vi "Begin.vi"() -> (1 "CameraDevRef":T5)   [LabVIEW 2011]
doc: "Called before other user functions, this VI is expected to open initial I/O refnums, load in file data, and do all program initialization. Notice that the <B>error out</B> terminal is simply used for data flow. Wiring it to other structures or subVIs ensures that this VI runs first."
uses:
  <vilib>/Rock Robotics/WPI/Camera/WPI_CameraDevRef.ctl
  <vilib>/Rock Robotics/WPI/Encoder/WPI_EncoderDevRef.ctl
  <vilib>/Rock Robotics/SystemInterfaces/Encoder/FPGA_EncoderIdx.ctl
  <vilib>/Rock Robotics/SystemInterfaces/Counter/FPGA_CounterCtrSystemIndex.ctl
  <vilib>/Rock Robotics/WPI/Encoder/WPI_EncoderType.ctl
  <vilib>/Rock Robotics/WPI/Joystick/WPI_JoystickDeviceEnum.ctl
  <vilib>/Rock Robotics/SystemInterfaces/DIO/FPGA_DIOPWMChannel.ctl
  <vilib>/Rock Robotics/SystemInterfaces/Typedef/FPGA_TypedefDigitalModule.ctl
  <vilib>/Rock Robotics/WPI/MotorControl/WPI_MotorControlOpen Victor.vi
  Robot Global Data.vi
  <vilib>/Rock Robotics/SystemInterfaces/DIO/FPGA_DIORelayChannel.ctl
  <vilib>/Rock Robotics/WPI/Relay/WPI_RelayDirection.ctl
  <vilib>/Rock Robotics/SystemInterfaces/AI/FPGA_AIChannel.ctl
  <vilib>/Rock Robotics/WPI/Counter/WPI_CounterDigitalInputToDigitalSource.vi
  <vilib>/Rock Robotics/SystemInterfaces/DIO/FPGA_DIOChannel.ctl
  <vilib>/Rock Robotics/SystemInterfaces/AI/FPGA_AIGyroChannel.ctl
  <vilib>/Rock Robotics/WPI/MotorControl/WPI_MotorControlOpen Jaguar.vi
  <vilib>/Rock Robotics/SystemInterfaces/Typedef/FPGA_TypedefAnalogModule.ctl
  <vilib>/Utility/file.llb/Read From Spreadsheet File (DBL).vi
panel:
  in  "Balls In Robot At Start":dbl=2.0
  out "LDriveEncoder 3":cluster{"status":bool}
  out "EncoderDevRef 3":T1={"DevStatus"={"status"=FALSE, "code"=0, "source"=""}, "EncoderIndex"=enum."Invalid", "CounterIndex"=enum."Invalid", "DistancePerCount"=1.0, "Decoding Type"=enum."4x"}
  out "EncoderDevRef 2":T1={"DevStatus"={"status"=FALSE, "code"=0, "source"=""}, "EncoderIndex"=enum."Invalid", "CounterIndex"=enum."Invalid", "DistancePerCount"=1.0, "Decoding Type"=enum."4x"}
  out "LDriveEncoder 2":errorcluster
  out "EncoderDevRef":T1={"DevStatus"={"status"=FALSE, "code"=0, "source"=""}, "EncoderIndex"=enum."Invalid", "CounterIndex"=enum."Invalid", "DistancePerCount"=1.0, "Decoding Type"=enum."4x"}
  out "LDriveEncoder":errorcluster
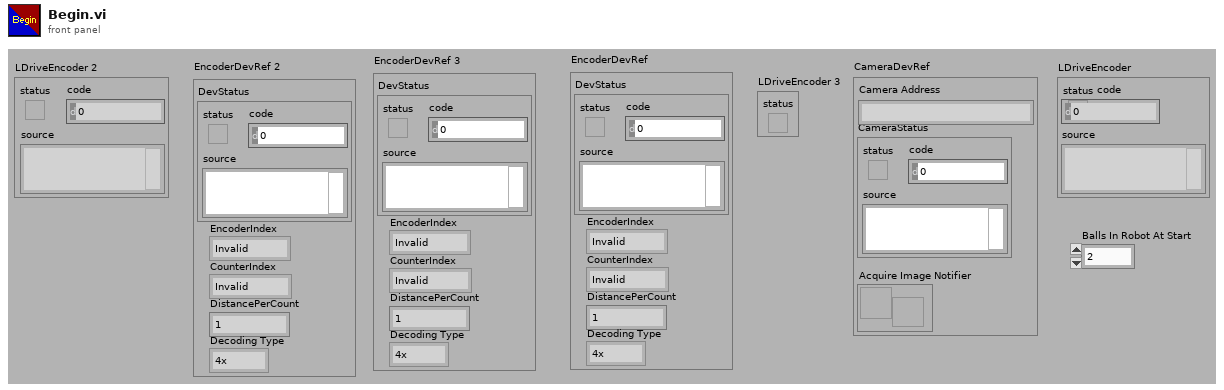
[diagram p1: front panel]
types:
  T1 = typedef "WPI_EncoderDevRef.ctl" = cluster{"DevStatus":errorcluster, "EncoderIndex":T2, "CounterIndex":T3, "DistancePerCount":dbl, "Decoding Type":T4}
  T2 = typedef "FPGA_EncoderIdx.ctl" = enum8{"Enc 0", "Enc 1", "Enc 2", "Enc 3", "Invalid"}
  T3 = typedef "FPGA_CounterCtrSystemIndex.ctl" = enum8{"Ctr 0", "Ctr 1", "Ctr 2", "Ctr 3", "Ctr 4", "Ctr 5", "Ctr 6", "Ctr 7", "Invalid"}
  T4 = typedef "WPI_EncoderType.ctl" = enum16{"1x", "2x", "4x"}
  T5 = typedef "WPI_CameraDevRef.ctl" = cluster{"Camera Address":string, "CameraStatus":errorcluster, "Acquire Image Notifier":refnum<notifier>}
  T6 = typedef "FPGA_TypedefDigitalModule.ctl" = enum16{"Digital Module 1", "Digital Module 2"}
  T7 = typedef "FPGA_DIOPWMChannel.ctl" = enum8{"PWM 1", "PWM 2", "PWM 3", "PWM 4", "PWM 5", "PWM 6", "PWM 7", "PWM 8", "PWM 9", "PWM 10", "Invalid"}
  T8 = typedef "WPI_JoystickDeviceEnum.ctl" = enum16{"USB 1", "USB 2", "USB 3", "USB 4", "Kinect 1", "Kinect 2"}
  T9 = typedef "FPGA_DIORelayChannel.ctl" = enum8{"Relay 1", "Relay 2", "Relay 3", "Relay 4", "Relay 5", "Relay 6", "Relay 7", "Relay 8", "Invalid"}
  T10 = typedef "FPGA_AIChannel.ctl" = enum8{"AI 1", "AI 2", "AI 3", "AI 4", "AI 5", "AI 6", "AI 7", "AI 8", "Invalid"}
  T11 = typedef "WPI_RelayDevRef.ctl" = cluster{"DevStatus":errorcluster, "Relay Channel":T9, "Digital Module":T6, "Relay Direction":T12}
  T12 = typedef "WPI_RelayDirection.ctl" = enum16{"Both directions", "Forward only", "Reverse only"}
  T13 = typedef "WPI_AnalogChannelDevRef.ctl" = cluster{"DevStatus":errorcluster, "Analog Module":T14, "Analog Channel":T10}
  T14 = typedef "FPGA_TypedefAnalogModule.ctl" = enum16{"Analog Module 1", "Analog Module 2"}
  T15 = typedef "WPI_MotorControlDeviceRef.ctl" = cluster{"DeviceStatus":errorcluster, "Type":enum16{"PWM", "CAN"}, "PWM":cluster{"Digital Module":T6, "PWM Channel":T7, "DeadBand":T16}, "CAN":cluster{"Device Number":u8, "Control Mode":T17, "Semaphore":T18, "Max Vout":dbl}, "Invert":bool, "TransformRef":T19, "InvTransformRef":T19}
  T16 = typedef "WPI_PWMDeadband.ctl" = cluster{"Name":string, "maxPositivePwm":i32, "minPositivePwm":i32, "centerPwm":i32, "maxNegativePwm":i32, "minNegativePwm":i32, "angularRange":u16}
  T17 = typedef "WPI_CANJaguar_ControlMode.ctl" = enum8{"Percent VBus", "Current", "Speed", "Position", "Voltage"}
  T18 = typedef "Semaphore RefNum" = refnum<k1>
  T19 = typedef "WPI_PWMTransform_ConPane.ctl" = refnum<vi>
  T20 = typedef "WPI_CameraImageSize.ctl" = enum16{"640x480", "320x240", "160x120"}
  T21 = cluster{"fps":i32, "compression":i32, "Image Size":T20}
  T22 = typedef "WPI_CameraWhite Balance Values.ctl" = enum16{"Auto", "Fixed indoor", "Fixed outdoor 1", "Fixed outdoor 2", "Fixed fluorescent 1", "Fixed fluorescent 2", "Hold current"}
  T23 = typedef "WPI_CameraExposure Values.ctl" = enum16{"Auto", "Flicker-free 50 Hz", "Flicker-free 60 Hz", "Hold current"}
  T24 = typedef "WPI_ServoDeviceRef.ctl" = cluster{"DeviceStatus":errorcluster, "Digital Module":T6, "PWM Channel":T7, "DeadBand":T16}
  T25 = typedef "FPGA_DIOChannel.ctl" = enum8{"DIO 1", "DIO 2", "DIO 3", "DIO 4", "DIO 5", "DIO 6", "DIO 7", "DIO 8", "DIO 9", "DIO 10", "DIO 11", "DIO 12", "DIO 13", "DIO 14", "Invalid"}
  T26 = typedef "WPI_DigitalInputDevRef.ctl" = cluster{"DevStatus":errorcluster, "DIO Channel":T25, "Digital Module":T6}
  T27 = typedef "FPGA_CounterEncoderSourceConvertionLVSourceType.ctl" = cluster{"DevStatus":errorcluster, "AnalogTriggerMode?":bool, "DigitalMode":cluster{"Digital Module":T6, "DIO Channel":T28}, "AnalogTriggerMode":cluster{"AnalogTriggerIndex":T29, "OutputType":T30}}
  T28 = typedef "FPGA_DIODigitalSourceChannel.ctl" = enum8{"DIO 1", "DIO 2", "DIO 3", "DIO 4", "DIO 5", "DIO 6", "DIO 7", "DIO 8", "DIO 9", "DIO 10", "DIO 11", "DIO 12", "DIO 13", "DIO 14", "Disabled"}
  T29 = typedef "FPGA_AnalogTriggerIndex.ctl" = enum8{"Trig 0", "Trig 1", "Trig 2", "Trig 3", "Trig 4", "Trig 5", "Trig 6", "Trig 7", "Invalid"}
  T30 = typedef "FPGA_AnalogTriggerOutType.ctl" = enum16{"InWindow", "TriggerState", "Rising", "Falling"}
  T31 = typedef "WPI_JoystickDevRef.ctl" = cluster{"Device":T8}
  T32 = typedef "FPGA_AIGyroChannel.ctl" = enum8{"AI 1", "AI 2", "Invalid"}
  T33 = typedef "WPI_GyroDevRef.ctl" = cluster{"DevStatus":errorcluster, "Analog Module":T14, "Analog Channel":T10, "Offset":dbl, "Gain (VoltsPerDegree/Second)":dbl}
  T34 = typedef "WPI_UltrasonicDeviceRef.ctl" = cluster{"DevStatus":errorcluster, "Ping Digital Module":T6, "Echo Digital Module":T6, "Ping Channel":T25, "Echo Channel":T25, "CntIndex":T3}
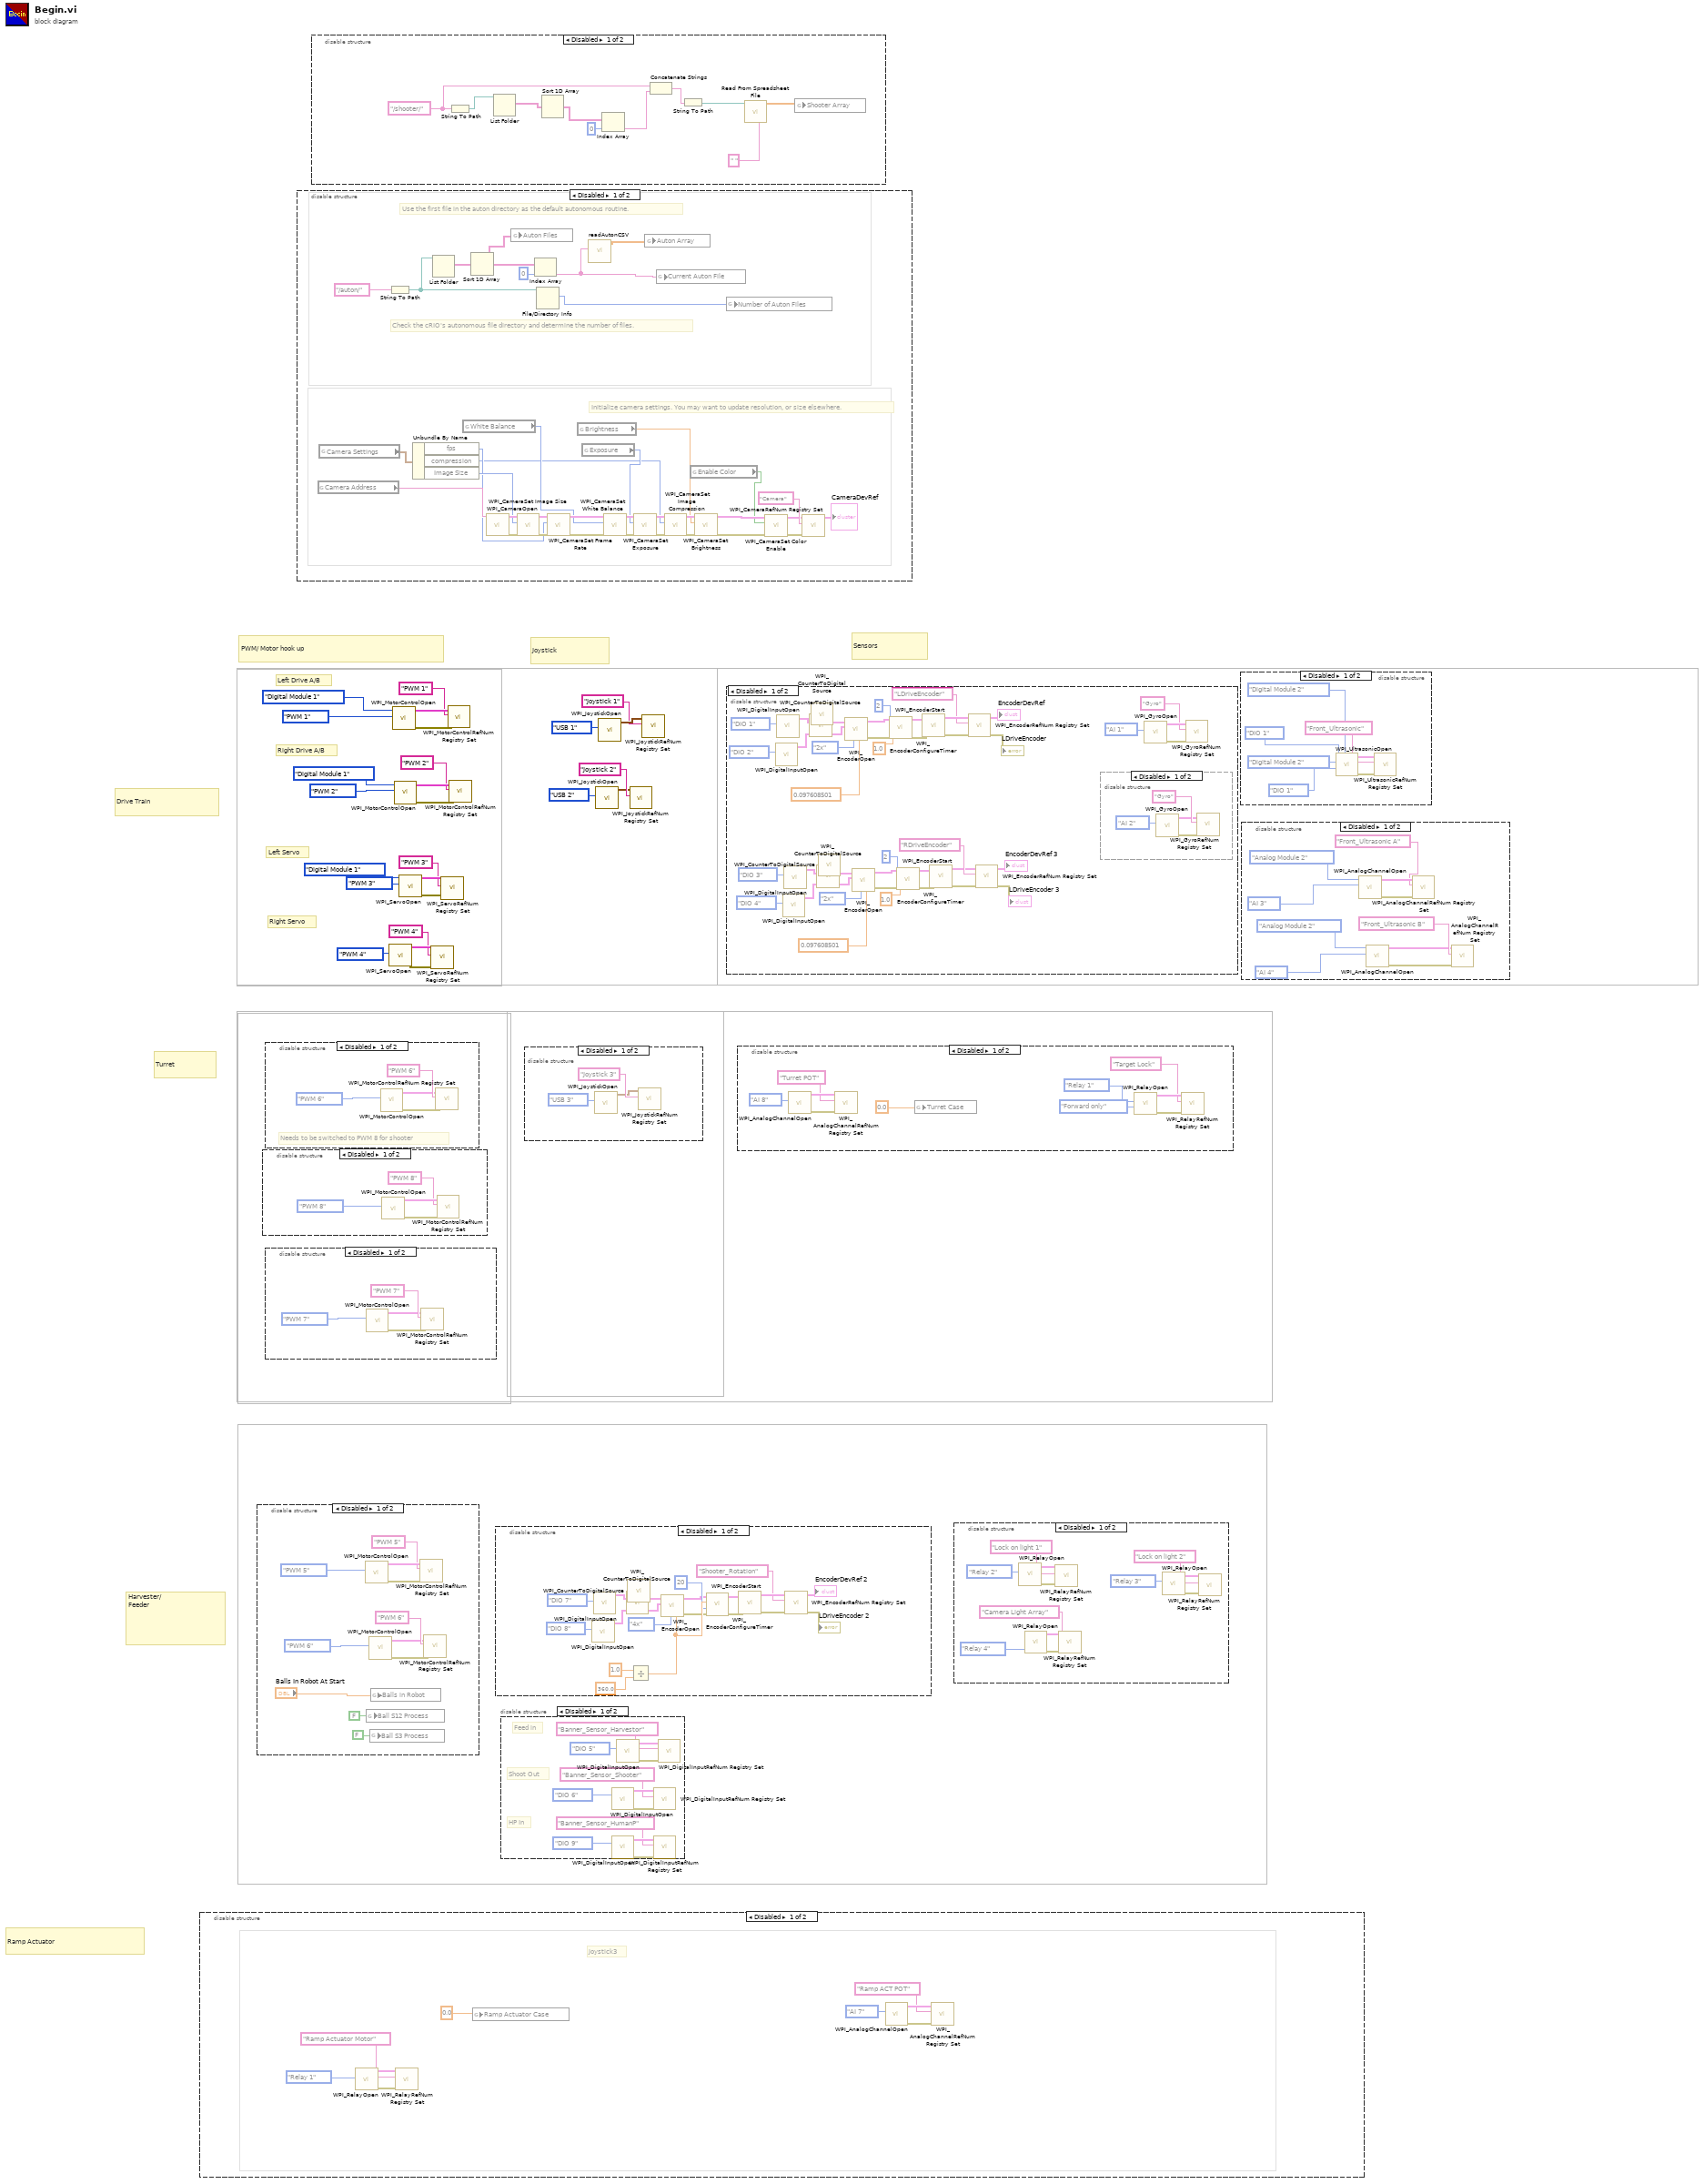
[diagram p0: block diagram]
diagram:
  # "Harvester/\nFeeder"
  # "Right Drive A/B"
  # "Left Drive A/B"
  # "Right Servo"
  # "Left Servo"
  # "Turret"
  # "Ramp Actuator"
  # "Drive Train"
  # "Sensors"
  # "Joystick"
  # "PWM/ Motor hook up"
  n1 = disable-structure shown="Disabled" {
    frame Disabled {
      # "Joystick3"
      n2 = call <vilib>:"WPI_RelayOpen.vi"("Relay Channel"=FPGA_DIORelayChannel."Relay 1") -> ("error out"=w30:errorcluster, "RelayDevRef"=w29:T11)  [unwired: 9 in]
      n3 = call <vilib>:"WPI_RelayRefNum Registry Set.vi"("error in (no error)"=w30, "refnum name"="Ramp Actuator Motor", "RelayDevRef"=w29) -> ()  [unwired: 7 in, 2 out]
      n4 = global write "Robot Global Data.vi" "Ramp Actuator Case"(0.0 ("Ramp Actuator Case")) -> ()
      n5 = call <vilib>:"WPI_AnalogChannelOpen.vi"("Analog Channel"=FPGA_AIChannel."AI 7") -> ("error out"=w33:errorcluster, "AIDeviceRef"=w34:T13)  [unwired: 9 in]
      n6 = call <vilib>:"WPI_AnalogChannelRefNum Registry Set.vi"("error in (no error)"=w33, "refnum name"="Ramp ACT POT", "AIDeviceRef"=w34) -> ()  [unwired: 7 in, 2 out]
    }
    frame Enabled {
    }
  }
  n7 = disable-structure shown="Disabled" {
    frame Disabled {
      n8 = call-poly <vilib>:"WPI_MotorControlOpen.vi"("PWM Channel"=FPGA_DIOPWMChannel."PWM 5") -> ("error out"=w42:errorcluster, "MotorControlDeviceRef"=w44:T15)  [unwired: 9 in]
      n9 = global write "Robot Global Data.vi" "Ball S12 Process"(FALSE ("Ball S12 Process")) -> ()
      n10 = call-poly <vilib>:"WPI_MotorControlOpen.vi"("PWM Channel"=FPGA_DIOPWMChannel."PWM 6") -> ("error out"=w41:errorcluster, "MotorControlDeviceRef"=w39:T15)  [unwired: 9 in]
      n11 = global write "Robot Global Data.vi" "Ball S3 Process"(FALSE ("Ball S3 Process")) -> ()
      n12 = global write "Robot Global Data.vi" "Balls in Robot"("Balls In Robot At Start") -> ()
      n13 = call <vilib>:"WPI_MotorControlRefNum Registry Set.vi"("error in (no error)"=w42, "refnum name"="PWM 5", "MotorControlDevRef"=w44) -> ()  [unwired: 7 in, 2 out]
      n14 = call <vilib>:"WPI_MotorControlRefNum Registry Set.vi"("error in (no error)"=w41, "refnum name"="PWM 6", "MotorControlDevRef"=w39) -> ()  [unwired: 7 in, 2 out]
    }
    frame Enabled {
    }
  }
  n15 = disable-structure shown="Disabled" {
    frame Disabled {
      n16 = call-poly <vilib>:"WPI_MotorControlOpen.vi"("PWM Channel"=FPGA_DIOPWMChannel."PWM 8") -> ("error out"=w46:errorcluster, "MotorControlDeviceRef"=w48:T15)  [unwired: 9 in]
      n17 = call <vilib>:"WPI_MotorControlRefNum Registry Set.vi"("error in (no error)"=w46, "refnum name"="PWM 8", "MotorControlDevRef"=w48) -> ()  [unwired: 7 in, 2 out]
    }
    frame Enabled {
    }
  }
  n18 = disable-structure shown="Disabled" {
    frame Disabled {
      # "Needs to be switched to PWM 8 for shooter"
      n19 = call-poly <vilib>:"WPI_MotorControlOpen.vi"("PWM Channel"=FPGA_DIOPWMChannel."PWM 6") -> ("error out"=w53:errorcluster, "MotorControlDeviceRef"=w51:T15)  [unwired: 9 in]
      n20 = call <vilib>:"WPI_MotorControlRefNum Registry Set.vi"("error in (no error)"=w53, "refnum name"="PWM 6", "MotorControlDevRef"=w51) -> ()  [unwired: 7 in, 2 out]
    }
    frame Enabled {
    }
  }
  n21 = disable-structure shown="Disabled" {
    frame Disabled {
      n22 = call-poly <vilib>:"WPI_MotorControlOpen.vi"("PWM Channel"=FPGA_DIOPWMChannel."PWM 7") -> ("error out"=w57:errorcluster, "MotorControlDeviceRef"=w55:T15)  [unwired: 9 in]
      n23 = call <vilib>:"WPI_MotorControlRefNum Registry Set.vi"("error in (no error)"=w57, "refnum name"="PWM 7", "MotorControlDevRef"=w55) -> ()  [unwired: 7 in, 2 out]
    }
    frame Enabled {
    }
  }
  n24 = disable-structure shown="Disabled" {
    frame Disabled {
      # "Check the cRIO's autonomous file directory and determine the number of files."
      # "Use the first file in the auton directory as the default autonomous routine."
      # "Initialize camera settings. You may want to update resolution, or size elsewhere."
      n25 = global read "Robot Global Data.vi" "Camera Address"() -> (w79:string)
      n26 = global read "Robot Global Data.vi" "Camera Settings"() -> (w78:T21)
      n27 = String To Path(string="/auton/") -> (path=w64:path)
      n28 = Unbundle By Name(w78) -> ("fps"=w76:i32, "compression"=w73:i32, "Image Size"=w77:T20)
      n29 = List Folder(path=w64) -> (filenames=w63:string[])  [unwired: 1 in, 5 out]
      n30 = global read "Robot Global Data.vi" "White Balance"() -> (w75:T22)
      n31 = Sort 1D Array(array=w63) -> (sorted array=w58:string[])
      n32 = call <vilib>:"WPI_CameraOpen.vi"("Camera Address"=w79) -> ("error out"=w85:errorcluster, "CameraDevRef"=w86:T5)  [unwired: 1 in, 8 out]
      n33 = global write "Robot Global Data.vi" "Auton Files"(w58) -> ()
      n34 = call <vilib>:"WPI_CameraSet Image Size.vi"("error in (no error)"=w85, "Image Size"=w77, "CameraDevRef"=w86) -> ("error out"=w84:errorcluster, "CameraDevRef Out"=w87:T5)  [unwired: 7 out]
      n35 = Index Array(array=w58, index=0) -> (element=w60:string)
      n36 = File/Directory Info(path=w64) -> (size=w61:i64)  [unwired: 1 in, 6 out]
      n37 = call <vilib>:"WPI_CameraSet Frame Rate.vi"("error in (no error)"=w84, "Frame Rate (fps)"=w76, "CameraDevRef"=w87) -> ("error out"=w83:errorcluster, "CameraDevRef Out"=w89:T5)  [unwired: 7 out]
      n38 = global read "Robot Global Data.vi" "Brightness"() -> (w72:dbl)
      n39 = global read "Robot Global Data.vi" "Exposure"() -> (w74:T23)
      n40 = call "readAutonCSV.vi"("AutonFile"=w60) -> ("AutonArray"=w59:dbl[][])  [unwired: 7 in]
      n41 = call <vilib>:"WPI_CameraSet White Balance.vi"("error in (no error)"=w83, "White Balance"=w75, "CameraDevRef"=w89) -> ("error out"=w82:errorcluster, "CameraDevRef Out"=w88:T5)  [unwired: 7 out]
      n42 = call <vilib>:"WPI_CameraSet Exposure.vi"("error in (no error)"=w82, "Exposure"=w74, "CameraDevRef"=w88) -> ("error out"=w81:errorcluster, "CameraDevRef Out"=w91:T5)  [unwired: 7 out]
      n43 = global write "Robot Global Data.vi" "Auton Array"(w59) -> ()
      n44 = global write "Robot Global Data.vi" "Current Auton File"(w60) -> ()
      n45 = call <vilib>:"WPI_CameraSet Image Compression.vi"("error in (no error)"=w81, "Compression"=w73, "CameraDevRef"=w91) -> ("error out"=w80:errorcluster, "CameraDevRef Out"=w90:T5)  [unwired: 7 out]
      n46 = global read "Robot Global Data.vi" "Enable Color"() -> (w67:bool)
      n47 = call <vilib>:"WPI_CameraSet Brightness.vi"("error in (no error)"=w80, "Brightness"=w72, "CameraDevRef"=w90) -> ("error out"=w70:errorcluster, "CameraDevRef Out"=w71:T5)  [unwired: 7 out]
      n48 = global write "Robot Global Data.vi" "Number of Auton Files"(w61) -> ()
      n49 = call <vilib>:"WPI_CameraSet Color Enable.vi"("error in (no error)"=w70, "Color Enabled"=w67, "CameraDevRef"=w71) -> ("error out"=w68:errorcluster, "CameraDevRef Out"=w69:T5)  [unwired: 7 in]
      n50 = call <vilib>:"WPI_CameraRefNum Registry Set.vi"("error in (no error)"=w68, "refnum name"="Camera", "CameraDevRef"=w69) -> ("CameraDevRef"=→"CameraDevRef":T5)  [unwired: 8 out]
    }
    frame Enabled {
    }
  }
  n51 = disable-structure shown="Disabled" {
    frame Disabled {
      w101 = "/shooter/" ("string")
      n52 = String To Path(string=w101) -> (path=w102:path)
      n53 = List Folder(path=w102) -> (filenames=w100:string[])  [unwired: 1 in, 5 out]
      n54 = Sort 1D Array(array=w100) -> (sorted array=w99:string[])
      n55 = Index Array(array=w99, index=0) -> (element=w97:string)
      n56 = Concatenate Strings(w101, w97) -> (w96:string)
      n57 = String To Path(string=w96) -> (path=w95:path)
      n58 = call-poly <vilib>:"Read From Spreadsheet File.vi"("delimiter (\\t)"=" " ("delimiter (\\t)"), "file path (dialog if empty)"=w95) -> ("all rows"=w93:dbl[][])  [unwired: 5 in, 4 out]
      n59 = global write "Robot Global Data.vi" "Shooter Array"(w93) -> ()
    }
    frame Enabled {
    }
  }
  n60 = call <vilib>:"WPI_ServoOpen.vi"("PWM Channel"=FPGA_DIOPWMChannel."PWM 4") -> ("error out"=w1:errorcluster, "ServoDeviceRef"=w16:T24)  [unwired: 9 in]
  n61 = call-poly <vilib>:"WPI_MotorControlOpen.vi"("PWM Channel"=FPGA_DIOPWMChannel."PWM 1", "Digital Module (Module 1)"=FPGA_TypedefDigitalModule."Digital Module 1") -> ("error out"=w6:errorcluster, "MotorControlDeviceRef"=w9:T15)  [unwired: 8 in]
  n62 = call-poly <vilib>:"WPI_MotorControlOpen.vi"("PWM Channel"=FPGA_DIOPWMChannel."PWM 2", "Digital Module (Module 1)"=FPGA_TypedefDigitalModule."Digital Module 1") -> ("error out"=w7:errorcluster, "MotorControlDeviceRef"=w12:T15)  [unwired: 8 in]
  n63 = call <vilib>:"WPI_ServoOpen.vi"("PWM Channel"=FPGA_DIOPWMChannel."PWM 3", "Digital Module (Module 1)"=FPGA_TypedefDigitalModule."Digital Module 1") -> ("error out"=w2:errorcluster, "ServoDeviceRef"=w18:T24)  [unwired: 8 in]
  n64 = call <vilib>:"WPI_ServoRefNum Registry Set.vi"("error in (no error)"=w1, "refnum name"="PWM 4", "ServoDeviceRef"=w16) -> ()  [unwired: 7 in, 2 out]
  n65 = call <vilib>:"WPI_ServoRefNum Registry Set.vi"("error in (no error)"=w2, "refnum name"="PWM 3", "ServoDeviceRef"=w18) -> ()  [unwired: 7 in, 2 out]
  n66 = call <vilib>:"WPI_MotorControlRefNum Registry Set.vi"("error in (no error)"=w6, "refnum name"="PWM 1", "MotorControlDevRef"=w9) -> ()  [unwired: 7 in, 2 out]
  n67 = call <vilib>:"WPI_MotorControlRefNum Registry Set.vi"("error in (no error)"=w7, "refnum name"="PWM 2", "MotorControlDevRef"=w12) -> ()  [unwired: 7 in, 2 out]
  n68 = disable-structure shown="Disabled" {
    frame Disabled {
      n69 = call <vilib>:"WPI_DigitalInputOpen.vi"("DIO Channel"=FPGA_DIOChannel."DIO 8") -> ("DigitalInputDevRef"=w107:T26)  [unwired: 9 in, 1 out]
      n70 = call <vilib>:"WPI_DigitalInputOpen.vi"("DIO Channel"=FPGA_DIOChannel."DIO 7") -> ("DigitalInputDevRef"=w104:T26)  [unwired: 9 in, 1 out]
      n71 = call-poly <vilib>:"WPI_CounterToDigitalSource.vi"("DigitalInputDevRef"=w107) -> ("Digital Source"=w108:T27)  [unwired: 6 in]
      n72 = call-poly <vilib>:"WPI_CounterToDigitalSource.vi"("DigitalInputDevRef"=w104) -> ("Digital Source"=w103:T27)  [unwired: 6 in]
      n73 = Divide(x=1.0, y=360.0) -> (x/y=w122:dbl)
      n74 = call <vilib>:"WPI_EncoderOpen.vi"("DistancePerCount"=w122, "Decoding Type"=WPI_EncoderType."4x", "BSource"=w108, "ASource"=w103) -> ("error out"=w111:errorcluster, "EncoderDevRef"=w112:T1)  [unwired: 6 in]
      n75 = call <vilib>:"WPI_EncoderConfigureTimer.vi"("error in (no error)"=w111, "Number Samples to Average"=u8 20, "Minimum Rate"=w122, "EncoderDevRef"=w112) -> ("error out"=w115:errorcluster, "EncoderDevRef"=w114:T1)  [unwired: 6 in]
      n76 = call <vilib>:"WPI_EncoderStart.vi"("error in (no error)"=w115, "EncoderDevRef"=w114) -> ("error out"=w117:errorcluster, "EncoderDevRef"=w116:T1)  [unwired: 8 in]
      n77 = call <vilib>:"WPI_EncoderRefNum Registry Set.vi"("error in (no error)"=w117, "refnum name"="Shooter_Rotation", "EncoderDevRef"=w116) -> ("error out"=→"LDriveEncoder 2":errorcluster, "EncoderDevRef"=→"EncoderDevRef 2":T1)  [unwired: 7 in]
    }
    frame Enabled {
    }
  }
  n78 = disable-structure shown="Disabled" {
    frame Disabled {
      # "HP In"
      # "Shoot Out"
      # "Feed in"
      n79 = call <vilib>:"WPI_DigitalInputOpen.vi"("DIO Channel"=FPGA_DIOChannel."DIO 6") -> ("error out"=w129:errorcluster, "DigitalInputDevRef"=w128:T26)  [unwired: 9 in]
      n80 = call <vilib>:"WPI_DigitalInputOpen.vi"("DIO Channel"=FPGA_DIOChannel."DIO 9") -> ("error out"=w125:errorcluster, "DigitalInputDevRef"=w124:T26)  [unwired: 9 in]
      n81 = call <vilib>:"WPI_DigitalInputOpen.vi"("DIO Channel"=FPGA_DIOChannel."DIO 5") -> ("error out"=w132:errorcluster, "DigitalInputDevRef"=w131:T26)  [unwired: 9 in]
      n82 = call <vilib>:"WPI_DigitalInputRefNum Registry Set.vi"("error in (no error)"=w129, "refnum name"="Banner_Sensor_Shooter", "DigitalInputDevRef"=w128) -> ()  [unwired: 7 in, 2 out]
      n83 = call <vilib>:"WPI_DigitalInputRefNum Registry Set.vi"("error in (no error)"=w125, "refnum name"="Banner_Sensor_HumanP", "DigitalInputDevRef"=w124) -> ()  [unwired: 7 in, 2 out]
      n84 = call <vilib>:"WPI_DigitalInputRefNum Registry Set.vi"("error in (no error)"=w132, "refnum name"="Banner_Sensor_Harvestor", "DigitalInputDevRef"=w131) -> ()  [unwired: 7 in, 2 out]
    }
    frame Enabled {
    }
  }
  n85 = disable-structure shown="Disabled" {
    frame Disabled {
      n86 = call <vilib>:"WPI_JoystickOpen.vi"("JoystickDevice"=WPI_JoystickDeviceEnum."USB 3") -> ("JoystickDevRef"=w136:T31)  [unwired: 10 in]
      n87 = call <vilib>:"WPI_JoystickRefNum Registry Set.vi"("refnum name"="Joystick 3", "JoystickDevRef"=w136) -> ()  [unwired: 8 in, 2 out]
    }
    frame Enabled {
    }
  }
  n88 = call <vilib>:"WPI_JoystickOpen.vi"("JoystickDevice"=WPI_JoystickDeviceEnum."USB 2") -> ("JoystickDevRef"=w22:T31)  [unwired: 10 in]
  n89 = call <vilib>:"WPI_JoystickOpen.vi"("JoystickDevice"=WPI_JoystickDeviceEnum."USB 1") -> ("JoystickDevRef"=w25:T31)  [unwired: 10 in]
  n90 = call <vilib>:"WPI_JoystickRefNum Registry Set.vi"("refnum name"="Joystick 2", "JoystickDevRef"=w22) -> ()  [unwired: 8 in, 2 out]
  n91 = call <vilib>:"WPI_JoystickRefNum Registry Set.vi"("refnum name"="Joystick 1", "JoystickDevRef"=w25) -> ()  [unwired: 8 in, 2 out]
  n92 = disable-structure shown="Disabled" {
    frame Disabled {
      n93 = call <vilib>:"WPI_DigitalInputOpen.vi"("DIO Channel"=FPGA_DIOChannel."DIO 2") -> ("DigitalInputDevRef"=w161:T26)  [unwired: 9 in, 1 out]
      n94 = call <vilib>:"WPI_DigitalInputOpen.vi"("DIO Channel"=FPGA_DIOChannel."DIO 1") -> ("DigitalInputDevRef"=w158:T26)  [unwired: 9 in, 1 out]
      n95 = call <vilib>:"WPI_DigitalInputOpen.vi"("DIO Channel"=FPGA_DIOChannel."DIO 4") -> ("DigitalInputDevRef"=w152:T26)  [unwired: 9 in, 1 out]
      n96 = call <vilib>:"WPI_DigitalInputOpen.vi"("DIO Channel"=FPGA_DIOChannel."DIO 3") -> ("DigitalInputDevRef"=w155:T26)  [unwired: 9 in, 1 out]
      n97 = call-poly <vilib>:"WPI_CounterToDigitalSource.vi"("DigitalInputDevRef"=w161) -> ("Digital Source"=w162:T27)  [unwired: 6 in]
      n98 = call-poly <vilib>:"WPI_CounterToDigitalSource.vi"("DigitalInputDevRef"=w158) -> ("Digital Source"=w157:T27)  [unwired: 6 in]
      n99 = call-poly <vilib>:"WPI_CounterToDigitalSource.vi"("DigitalInputDevRef"=w152) -> ("Digital Source"=w151:T27)  [unwired: 6 in]
      n100 = call-poly <vilib>:"WPI_CounterToDigitalSource.vi"("DigitalInputDevRef"=w155) -> ("Digital Source"=w156:T27)  [unwired: 6 in]
      n101 = call <vilib>:"WPI_EncoderOpen.vi"("DistancePerCount"=0.097608501, "Decoding Type"=WPI_EncoderType."2x", "BSource"=w162, "ASource"=w157) -> ("error out"=w166:errorcluster, "EncoderDevRef"=w167:T1)  [unwired: 6 in]
      n102 = call <vilib>:"WPI_EncoderOpen.vi"("DistancePerCount"=0.097608501, "Decoding Type"=WPI_EncoderType."2x", "BSource"=w151, "ASource"=w156) -> ("error out"=w147:errorcluster, "EncoderDevRef"=w146:T1)  [unwired: 6 in]
      n103 = call <vilib>:"WPI_EncoderConfigureTimer.vi"("error in (no error)"=w166, "Number Samples to Average"=u8 2, "Minimum Rate"=1.0, "EncoderDevRef"=w167) -> ("error out"=w171:errorcluster, "EncoderDevRef"=w170:T1)  [unwired: 6 in]
      n104 = call <vilib>:"WPI_EncoderConfigureTimer.vi"("error in (no error)"=w147, "Number Samples to Average"=u8 2, "Minimum Rate"=1.0, "EncoderDevRef"=w146) -> ("error out"=w142:errorcluster, "EncoderDevRef"=w143:T1)  [unwired: 6 in]
      n105 = call <vilib>:"WPI_EncoderStart.vi"("error in (no error)"=w171, "EncoderDevRef"=w170) -> ("error out"=w173:errorcluster, "EncoderDevRef"=w172:T1)  [unwired: 8 in]
      n106 = call <vilib>:"WPI_EncoderStart.vi"("error in (no error)"=w142, "EncoderDevRef"=w143) -> ("error out"=w140:errorcluster, "EncoderDevRef"=w141:T1)  [unwired: 8 in]
      n107 = call <vilib>:"WPI_EncoderRefNum Registry Set.vi"("error in (no error)"=w173, "refnum name"="LDriveEncoder", "EncoderDevRef"=w172) -> ("error out"=→"LDriveEncoder":errorcluster, "EncoderDevRef"=→"EncoderDevRef":T1)  [unwired: 7 in]
      n108 = call <vilib>:"WPI_EncoderRefNum Registry Set.vi"("error in (no error)"=w140, "refnum name"="RDriveEncoder", "EncoderDevRef"=w141) -> ("error out"=→"LDriveEncoder 3":errorcluster, "EncoderDevRef"=→"EncoderDevRef 3":T1)  [unwired: 7 in]
      n109 = disable-structure shown="Disabled" {
        frame Disabled {
          n110 = call <vilib>:"WPI_GyroOpen.vi"("Analog Channel"=FPGA_AIGyroChannel."AI 2") -> ("error out"=w180:errorcluster, "GyroDevRef"=w181:T33)  [unwired: 8 in, 1 out]
          n111 = call <vilib>:"WPI_GyroRefNum Registry Set.vi"("error in (no error)"=w180, "refnum name"="Gyro", "GyroDevRef"=w181) -> ()  [unwired: 7 in, 2 out]
        }
        frame Enabled {
        }
      }
      n112 = call <vilib>:"WPI_GyroOpen.vi"("Analog Channel"=FPGA_AIGyroChannel."AI 1") -> ("error out"=w179:errorcluster, "GyroDevRef"=w178:T33)  [unwired: 8 in, 1 out]
      n113 = call <vilib>:"WPI_GyroRefNum Registry Set.vi"("error in (no error)"=w179, "refnum name"="Gyro", "GyroDevRef"=w178) -> ()  [unwired: 7 in, 2 out]
    }
    frame Enabled {
    }
  }
  n114 = disable-structure shown="Disabled" {
    frame Disabled {
      n115 = call <vilib>:"WPI_AnalogChannelOpen.vi"("Analog Channel"=FPGA_AIChannel."AI 8") -> ("error out"=w187:errorcluster, "AIDeviceRef"=w188:T13)  [unwired: 9 in]
      n116 = call <vilib>:"WPI_AnalogChannelRefNum Registry Set.vi"("error in (no error)"=w187, "refnum name"="Turret POT", "AIDeviceRef"=w188) -> ()  [unwired: 7 in, 2 out]
      n117 = global write "Robot Global Data.vi" "Turret Case"(0.0 ("Return To Home Case")) -> ()
      n118 = call <vilib>:"WPI_RelayOpen.vi"("Relay Direction"=WPI_RelayDirection."Forward only", "Relay Channel"=FPGA_DIORelayChannel."Relay 1") -> ("error out"=w192:errorcluster, "RelayDevRef"=w193:T11)  [unwired: 8 in]
      n119 = call <vilib>:"WPI_RelayRefNum Registry Set.vi"("error in (no error)"=w192, "refnum name"="Target Lock", "RelayDevRef"=w193) -> ()  [unwired: 7 in, 2 out]
    }
    frame Enabled {
    }
  }
  n120 = disable-structure shown="Disabled" {
    frame Disabled {
      n121 = call <vilib>:"WPI_RelayOpen.vi"("Relay Channel"=FPGA_DIORelayChannel."Relay 2") -> ("error out"=w203:errorcluster, "RelayDevRef"=w202:T11)  [unwired: 9 in]
      n122 = call <vilib>:"WPI_RelayOpen.vi"("Relay Channel"=FPGA_DIORelayChannel."Relay 4") -> ("error out"=w205:errorcluster, "RelayDevRef"=w204:T11)  [unwired: 9 in]
      n123 = call <vilib>:"WPI_RelayRefNum Registry Set.vi"("error in (no error)"=w203, "refnum name"="Lock on light 1", "RelayDevRef"=w202) -> ()  [unwired: 7 in, 2 out]
      n124 = call <vilib>:"WPI_RelayRefNum Registry Set.vi"("error in (no error)"=w205, "refnum name"="Camera Light Array", "RelayDevRef"=w204) -> ()  [unwired: 7 in, 2 out]
      n125 = call <vilib>:"WPI_RelayOpen.vi"("Relay Channel"=FPGA_DIORelayChannel."Relay 3") -> ("error out"=w194:errorcluster, "RelayDevRef"=w195:T11)  [unwired: 9 in]
      n126 = call <vilib>:"WPI_RelayRefNum Registry Set.vi"("error in (no error)"=w194, "refnum name"="Lock on light 2", "RelayDevRef"=w195) -> ()  [unwired: 7 in, 2 out]
    }
    frame Enabled {
    }
  }
  n127 = disable-structure shown="Disabled" {
    frame Disabled {
      n128 = call <vilib>:"WPI_UltrasonicOpen.vi"("Ping Digital Module (Module 1)"=FPGA_TypedefDigitalModule."Digital Module 2", "Echo DIO Channel"=FPGA_DIOChannel."DIO 1", "Echo Digital Module (Module 1)"=FPGA_TypedefDigitalModule."Digital Module 2", "Ping DIO Channel"=FPGA_DIOChannel."DIO 1") -> ("error out"=w212:errorcluster, "UltrasonicDevRef"=w211:T34)  [unwired: 6 in]
      n129 = call <vilib>:"WPI_UltrasonicRefNum Registry Set.vi"("error in (no error)"=w212, "refnum name"="Front_Ultrasonic", "UltrasonicDevRef"=w211) -> ()  [unwired: 7 in, 2 out]
    }
    frame Enabled {
    }
  }
  n130 = disable-structure shown="Disabled" {
    frame Disabled {
      n131 = call <vilib>:"WPI_AnalogChannelOpen.vi"("Analog Channel"=FPGA_AIChannel."AI 3", "Analog Module (Module 1)"=FPGA_TypedefAnalogModule."Analog Module 2") -> ("error out"=w218:errorcluster, "AIDeviceRef"=w217:T13)  [unwired: 8 in]
      n132 = call <vilib>:"WPI_AnalogChannelOpen.vi"("Analog Channel"=FPGA_AIChannel."AI 4", "Analog Module (Module 1)"=FPGA_TypedefAnalogModule."Analog Module 2") -> ("error out"=w213:errorcluster, "AIDeviceRef"=w214:T13)  [unwired: 8 in]
      n133 = call <vilib>:"WPI_AnalogChannelRefNum Registry Set.vi"("error in (no error)"=w218, "refnum name"="Front_Ultrasonic A", "AIDeviceRef"=w217) -> ()  [unwired: 7 in, 2 out]
      n134 = call <vilib>:"WPI_AnalogChannelRefNum Registry Set.vi"("error in (no error)"=w213, "refnum name"="Front_Ultrasonic B", "AIDeviceRef"=w214) -> ()  [unwired: 7 in, 2 out]
    }
    frame Enabled {
    }
  }
